vi "merFISH_sort_laser_lines.vi"(4 "Laser lines array":dbl[][](array[numeric])) -> (0 "Laser lines photobleaching":dbl[][](array[numeric]), 1 "Laser lines merFISH":dbl[][](array[numeric]), 2 "N laser lines merFISH":i32)   [LabVIEW 2015]
panel:
  out "N laser lines photobleaching":i32
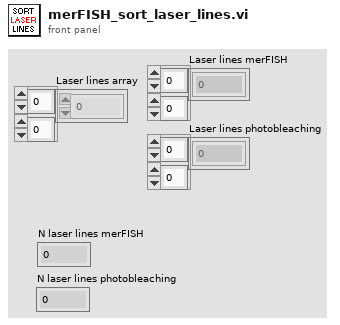
[diagram p1: front panel]
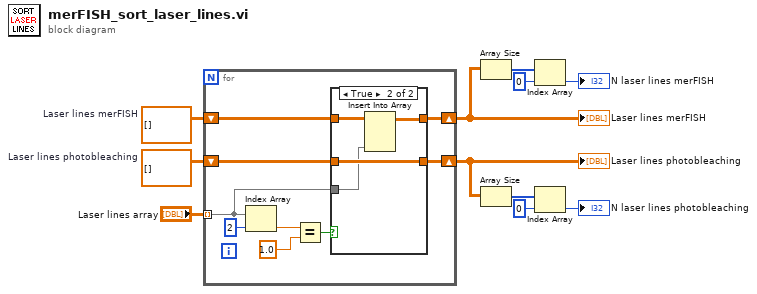
[diagram p0: block diagram]
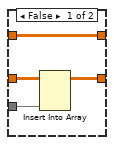
[diagram p2: hidden frame]
diagram:
  w9 = dbl[][] []  # Laser lines photobleaching
  w10 = dbl[][] []  # Laser lines merFISH
  n1 = for {
    tunnel: "Laser lines array" -> [w13] mode=indexing
    shift-right: [w12] -> w1
    shift-left: w9 -> [w16]
    shift-right: [w14] -> w8
    shift-left: w10 -> [w15]
    n2 = Index Array(array=w13, index=2) -> (element=w19:dbl)
    n3 = Equal?(x=w19, y=1.0) -> (x = y?=w17:bool)
    n4 = case shown="True" w17 {
      tunnel: w16 -> [w23 w28]
      tunnel: w15 -> [w24 w27]
      tunnel: [w24 w26] -> w14
      tunnel: w13 -> [w22 w25]
      tunnel: [w21 w28] -> w12
      frame False {
        n5 = Insert Into Array(array=w23, new element=w22) -> (w21:dbl[][])  [unwired: 2 in]
      }
      frame True {
        n6 = Insert Into Array(array=w27, new element=w25) -> (w26:dbl[][])  [unwired: 2 in]
      }
    }
  }
  "Laser lines merFISH" <- w8
  "Laser lines photobleaching" <- w1
  n7 = Array Size(array=w8) -> (size(s)=w7:i32[])
  n8 = Array Size(array=w1) -> (size(s)=w2:i32[])
  n9 = Index Array(array=w7, index=0) -> (element=→"N laser lines merFISH":i32)
  n10 = Index Array(array=w2, index=0) -> (element=→"N laser lines photobleaching":i32)
